vi "Read Settings.vi"(8 "error in (no error)":errorcluster, 11 "ProgramSettings in":refnum<class "ProgramSettings.lvclass">) -> (0 "error out":errorcluster, 2 "Settings":T1={"Serial Port for strømforsyning"="COM12", "Serial Port for SSI Interface"="COM12"}, 3 "ProgramSettings out":refnum<class "ProgramSettings.lvclass">)   [LabVIEW 2019, in "ProgramSettings.lvclass"]
uses:
  ProgramSettings.lvclass
  ProgramSettings.lvclass/ProgramSettings.ctl
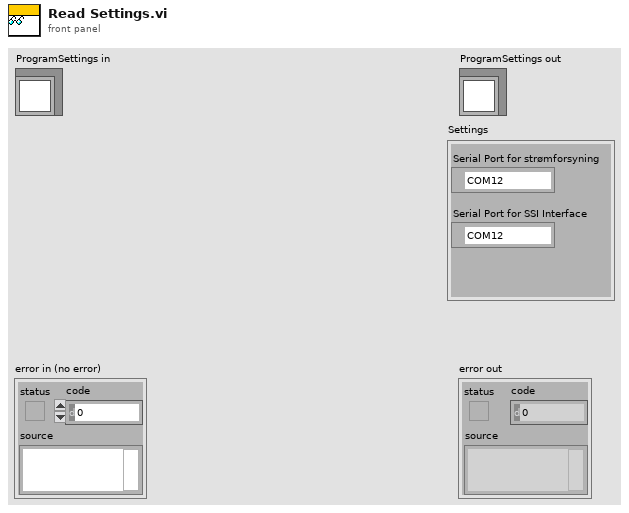
[diagram p1: front panel]
types:
  T1 = cluster{"Serial Port for strømforsyning":refnum<visa-resource-name>, "Serial Port for SSI Interface":refnum<visa-resource-name>}
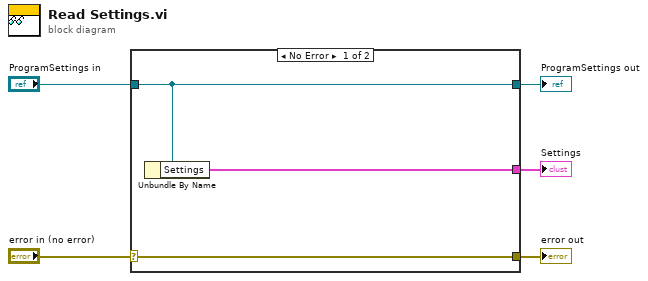
[diagram p0: block diagram]
diagram:
  n1 = case shown="No Error" "error in (no error)" {
    selector: "error in (no error)" -> [w8 w9]
    tunnel: [w8 w9] -> w4
    tunnel: [w7 w10] -> w2
    tunnel: "ProgramSettings in" -> [w7 w10]
    tunnel: [w6 _] -> w1
    frame No Error {
      n2 = Unbundle By Name(w7) -> ("Settings"=w6:T1)
    }
    frame Error {
    }
  }
  "error out" <- w4
  "ProgramSettings out" <- w2
  "Settings" <- w1
